vi "Vector joystck.vi"(0 "Jx input":dbl=1.0 min=-1.0 max=1.0 format="%.4f", 5 "Jy input":dbl=0.04 min=-1.0 max=1.0 format="%.4f", 7 "Jr input":dbl=1.0 min=-1.0 max=1.0 format="%.4f") -> (4 "Jx":dbl=0.9992009587217894 format="%#.4f", 6 "Jy":dbl format="%#.4f", 8 "Jr":dbl=1.0 format="%#.4f", 10 "R":dbl=1.0, 13 "theta (deg)":dbl=2.29061004263853, 14 "theta (rad)":dbl=0.039978687123290044)   [LabVIEW 2023]
uses:
  <vilib>/Analysis/coordinate.llb/Angle Units.ctl
  <vilib>/Analysis/coordinate.llb/Angle Range (Degree).ctl
  <vilib>/Analysis/coordinate.llb/Wrap Angle (scalar).vi
  <vilib>/Analysis/NI_AAL_Angle.lvlib
panel:
  out "XY after\nDEADBAND":cluster{"X":dbl, "Y":dbl}={"X"=1.0, "Y"=0.04}
  in  "resting steer angle (deg)":dbl=90.0 format="%#_13g"
  in  "Reset":bool
  in  "axis dead band":dbl=0.05000000000000004 format="%#_13g"
  in  "Max dx/dt":dbl=10.0
  out "Joystick":cluster{dbl[], dbl[]}(graph)={[0.0, 1.0], [0.0, 0.04]}
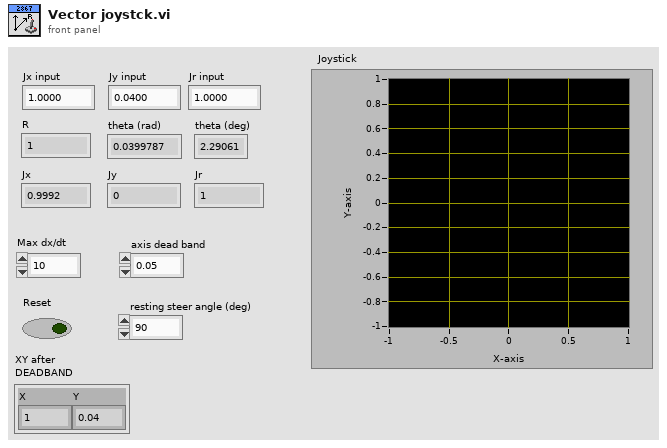
[diagram p1: front panel]
types:
  T1 = typedef "NI_AAL_Angle.lvlib/Angle Range (Degree).ctl" = u16
  T2 = typedef "NI_AAL_Angle.lvlib/Angle Units.ctl" = i32
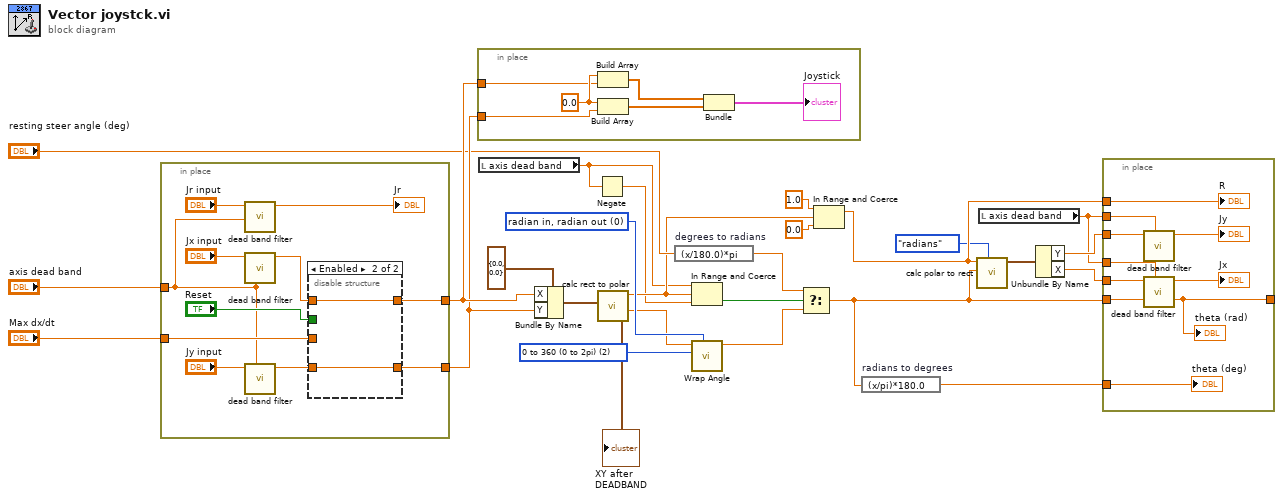
[diagram p0: block diagram]
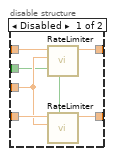
[diagram p2: hidden frame]
diagram:
  w13 = T1 2 items=["none", "-180 to 180 (-pi to pi)", "0 to 360 (0 to 2pi)"] ("angle range")
  w14 = T2 0 items=["radian in, radian out", "radian in, degree out", "degree in, degree out", "degree in, radian out"] ("angle units")
  n1 = in-place {
    in-place-border: [w34] -> w21
    in-place-border: [w33] -> w20
    in-place-border: "Max dx/dt" -> [w31]
    in-place-border: "axis dead band" -> [w28]
    n2 = call "dead band filter.vi"("deadband"=w28, "input"="Jr input") -> ("output"=→"Jr":dbl)  [unwired: 9 in]
    n3 = call "dead band filter.vi"("deadband"=w28, "input"="Jx input") -> ("output"=w35:dbl)  [unwired: 9 in]
    n4 = call "dead band filter.vi"("deadband"=w28, "input"="Jy input") -> ("output"=w32:dbl)  [unwired: 9 in]
    n5 = disable-structure shown="Enabled" {
      disable-tunnel: w35 -> [w43 w45]
      disable-tunnel: [w42 w45] -> w34
      disable-tunnel: [w41 w44] -> w33
      disable-tunnel: w32 -> [w40 w44]
      disable-tunnel: w31 -> [w39 _]
      disable-tunnel: "Reset" -> [w38 _]
      frame Disabled {
        n6 = call "RateLimiter.vi"("Reset"=w38, "Max dx/dt"=w39, "Input"=w43) -> ("Output"=w42:dbl)  [unwired: 8 in]
        n7 = call "RateLimiter.vi"("Reset"=w38, "Max dx/dt"=w39, "Input"=w40) -> ("Output"=w41:dbl)  [unwired: 8 in]
      }
      frame Enabled {
      }
    }
  }
  n8 = in-place {
    in-place-border: w21 -> [w50]
    in-place-border: w20 -> [w49]
    w51 = 0.0 ("element")
    n9 = Build Array(w51, w50) -> (w47:dbl[])
    n10 = Build Array(w51, w49) -> (w46:dbl[])
    n11 = Bundle(w47, w46) -> (→"Joystick":cluster{dbl[], dbl[]})  [unwired: 1 in]
  }
  n12 = local read "axis dead band"() -> (w3:dbl)
  n13 = Bundle By Name(cluster=cluster{"X":dbl, "Y":dbl} {"X"=0.0, "Y"=0.0} ("XY"), "X"=w21, "Y"=w20) -> (w7:cluster{"X":dbl, "Y":dbl})
  "XY after\nDEADBAND" <- w7
  n14 = Negate(x=w3) -> (-x=w2:dbl)
  n15 = call "calc rect to polar.vi"("XY"=w7) -> ("angle (rad)"=w9:dbl, "Magnitude"=w10:dbl)  [unwired: 8 in, 1 out]
  n16 = expression code="(x/180.0)*pi" "degrees to radians"("resting steer angle (deg)") -> (w4:dbl)
  n17 = In Range and Coerce(upper limit=w3, x=w10, lower limit=w2) -> (In Range?=w11:bool)  [unwired: 1 out]
  n18 = call-poly <vilib>:"Wrap Angle.vi"("angle units"=w14, "angle range"=w13, "angle in"=w9) -> ("angle out"=w6:dbl)  [unwired: 7 in, 1 out]
  n19 = Select(t=w4, s=w11, f=w6) -> (s? t:f=w23:dbl)
  n20 = In Range and Coerce(upper limit=1.0, x=w10, lower limit=0.0 ("x")) -> (coerced(x)=w22:dbl)  [unwired: 1 out]
  n21 = expression code="(x/pi)*180.0" "radians to degrees"(w23) -> (w24:dbl)
  n22 = call "calc polar to rect.vi"("units"=enum16{"degrees", "radians"}."radians", "angle"=w23, "mag"=w22) -> ("XY"=w15:cluster{"X":dbl, "Y":dbl})  [unwired: 8 in]
  n23 = local read "axis dead band"() -> (w1:dbl)
  n24 = Unbundle By Name(w15) -> ("Y"=w25:dbl, "X"=w26:dbl)
  n25 = in-place {
    in-place-border: w26 -> [w58]
    in-place-border: w25 -> [w56]
    in-place-border: w24 -> [w60]
    in-place-border: w23 -> [w54]
    in-place-border: w22 -> [w59]
    in-place-border: [w54] -> _
    in-place-border: w1 -> [w53]
    in-place-border: w1 -> [w52]
    n26 = call "dead band filter.vi"("deadband"=w53, "input"=w56) -> ("output"=→"Jy":dbl)  [unwired: 9 in]
    n27 = call "dead band filter.vi"("deadband"=w52, "input"=w58) -> ("output"=→"Jx":dbl)  [unwired: 9 in]
    "theta (deg)" <- w60
    "theta (rad)" <- w54
    "R" <- w59
  }
